vi "Execute Command.vi"(8 "error in (no error)":errorcluster, 10 "Command In":refnum<class "Command.lvclass">, 11 "Command Processor in":refnum<class "Command Processor.lvclass">) -> (0 "error out":errorcluster, 3 "Command Processor out":refnum<class "Command Processor.lvclass">)   [LabVIEW 2013, in "Command Processor.lvlib" / "Command Processor.lvclass"]
uses:
  Command Processor.lvclass
  Command/Command.lvclass
  <vilib>/ActorFramework/Actor/Actor.lvclass/Actor.ctl
  <vilib>/ActorFramework/Message Enqueuer/Message Enqueuer.lvclass/Message Enqueuer.ctl
  Command Processor.lvclass/Command Processor.ctl
  <vilib>/ActorFramework/Message Enqueuer/Init from Existing Queue.vi
  <vilib>/ActorFramework/Message Enqueuer/Enqueue.vi
  <vilib>/ActorFramework/Message Priority Queue/Priority Enqueue.vi
  <vilib>/ActorFramework/Message Enqueuer/Message Enqueuer.lvclass
  Command Messages/Start Msg/Start Command Msg.lvclass
  <vilib>/ActorFramework/Actor/Actor.lvclass
  Command Processor Messages/Go To Executing Msg/Go To Executing Msg.lvclass
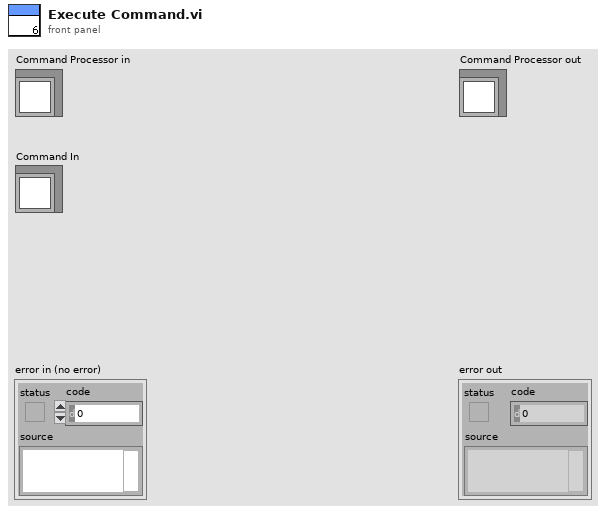
[diagram p1: front panel]
types:
  T1 = typedef "Command Processor.lvlib/Command Processor.lvclass/Command Processor Status.ctl" = cluster{"State Entry time":timestamp, "State Status":T2, "Command Processor Current State":string, "Command Status":T4}
  T2 = typedef "Current Previous State Status.ctl" = cluster{"Current State Status":T3, "Previous State Status":T3}
  T3 = typedef "State Status.ctl" = cluster{"State Name":string, "State Entry Time":timestamp, "State Exit Time":timestamp}
  T4 = typedef "Command Processor.lvlib/Command.lvlib/Command.lvclass/Command Status.ctl" = cluster{"Command Name":string, "Current State Status":T5, "Command Start Time":timestamp, "Command End Time":timestamp, "Previous State Status":T5}
  T5 = typedef "Command Processor.lvlib/Command.lvlib/Command.lvclass/State Status.ctl" = cluster{"State Name":string, "State Entry Time":timestamp, "State Exit Time":timestamp}
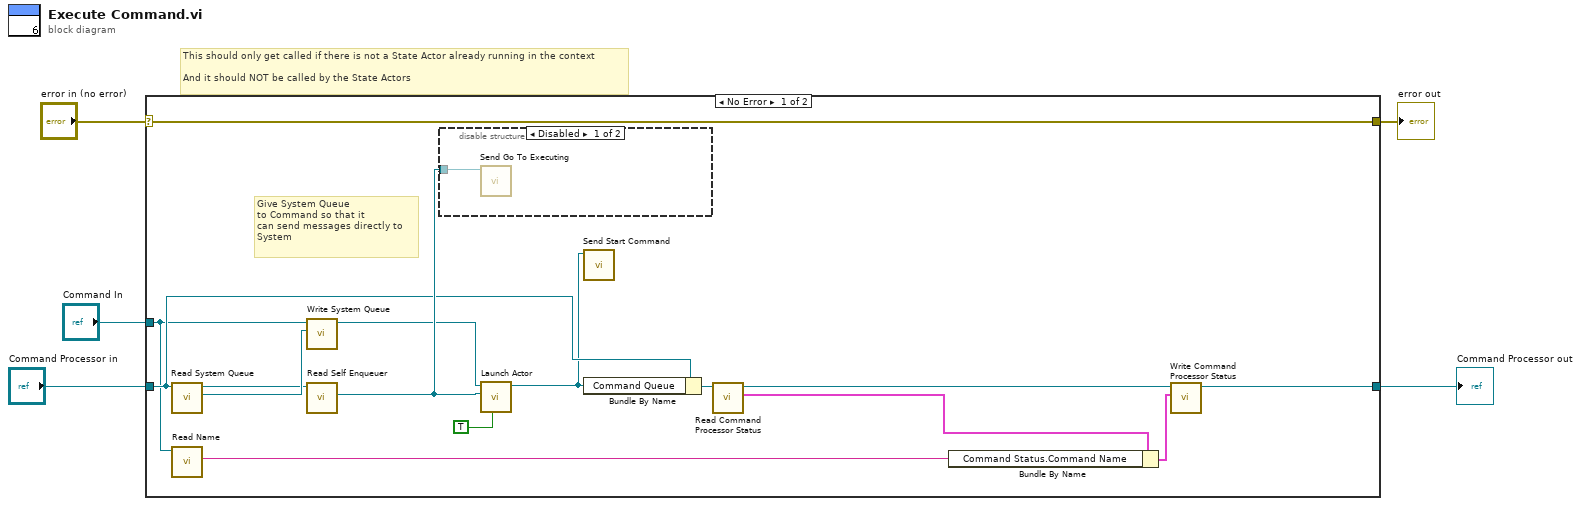
[diagram p0: block diagram]
diagram:
  # "This should only get called if there is not a State Actor already running in the context\n\nAnd it should NOT be called by the State Actors"
  n1 = case shown="No Error" "error in (no error)" {
    selector: "error in (no error)" -> [w20 w23]
    tunnel: [w20 w23] -> w4
    tunnel: [w16 w22] -> w2
    tunnel: "Command Processor in" -> [w11 w22]
    tunnel: "Command In" -> [w10 _]
    frame No Error {
      # "Give System Queue \nto Command so that it\ncan send messages directly to \nSystem"
      n2 = call-dynamic "Read System Queue.vi"("Command Processor in"=w11) -> ("System Queue"=w8:refnum<class "Message Enqueuer.lvclass">, "Command Processor out"=w7:refnum<class "Command Processor.lvclass">)  [unwired: 8 in, 1 out]
      n3 = call-dynamic "Read Name.vi"("Command in"=w10) -> ("Name"=w13:string)  [unwired: 8 in, 2 out]
      n4 = call-dynamic "Write System Queue.vi"("Actor Framework:Message Enqueuer"=w8, "Command in"=w10) -> ("Command out"=w9:refnum<class "Command.lvclass">)  [unwired: 8 in, 1 out]
      n5 = call <vilib>:"Read Self Enqueuer.vi"("Actor"=w7) -> ("Self Enqueuer"=w12:refnum<class "Message Enqueuer.lvclass">)  [unwired: 10 in]
      n6 = disable-structure shown="Disabled" {
        disable-tunnel: w12 -> [w21 _]
        frame Disabled {
          n7 = call "Send Go To Executing.vi"("Message Enqueuer"=w21) -> ()  [unwired: 9 in, 2 out]
        }
        frame Enabled {
        }
      }
      n8 = call <vilib>:"Launch Actor.vi"("Open Actor Core front panel? (F)"=TRUE, "Actor-to-Caller Enqueuer"=w12, "Actor"=w9) -> ("Caller-To-Actor Enqueuer"=w6:refnum<class "Message Enqueuer.lvclass">)  [unwired: 7 in, 1 out]
      n9 = call "Send Start Command.vi"("Message Enqueuer"=w6) -> ()  [unwired: 9 in, 2 out]
      n10 = Bundle By Name(cluster=w11, "Command Queue"=w6) -> (w18:refnum<class "Command Processor.lvclass">)
      n11 = call-dynamic "Read Command Processor Status.vi"("Command Processor in"=w18) -> ("Command Processor Status"=w15:T1, "Command Processor out"=w17:refnum<class "Command Processor.lvclass">)  [unwired: 8 in, 1 out]
      n12 = Bundle By Name(cluster=w15, "Command Status.Command Name"=w13) -> (w14:T1)
      n13 = call-dynamic "Write Command Processor Status.vi"("Command Processor Status"=w14, "Command Processor in"=w17) -> ("Command Processor out"=w16:refnum<class "Command Processor.lvclass">)  [unwired: 8 in, 1 out]
    }
    frame Error {
    }
  }
  "error out" <- w4
  "Command Processor out" <- w2
